vi "Initialize Subpanel Objects.vi"(8 "error in (no error)":errorcluster, 10 "SubPanelRefs":refnum<vi>[](array[refnum]), 11 "HSplittedX2 in":refnum<class "HSplittedX2.lvclass">) -> (0 "error out":errorcluster, 3 "HSplittedX2 out":refnum<class "HSplittedX2.lvclass">)   [LabVIEW 2020, in "HSplittedX2.lvlib" / "HSplittedX2.lvclass"]
uses:
  HSplittedX2.lvclass
  HSplittedX2.lvclass/HSplittedX2.ctl
  <vilib>/MGI/Panel Manager/Panel/Panel.lvlib
  <vilib>/MGI/Panel Manager/Panel/Panel/Subpanel/Subpanel.vi
  <vilib>/MGI/Panel Manager/Panel/Panel/Subpanel/Subpanel.lvclass
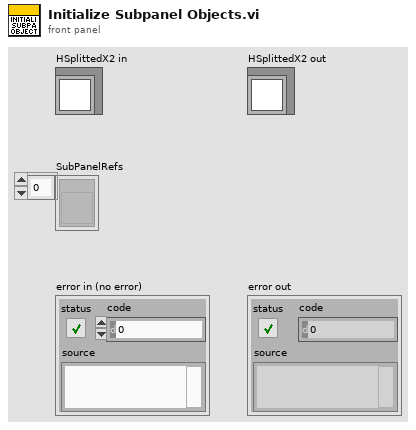
[diagram p1: front panel]
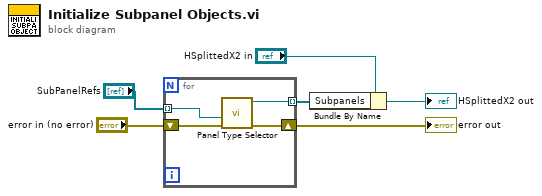
[diagram p0: block diagram]
diagram:
  n1 = for {
    tunnel: "SubPanelRefs" -> [w10] mode=indexing
    tunnel: [w9] -> w4 mode=indexing
    shift-right: [w7] -> w6
    shift-left: "error in (no error)" -> [w8]
    n2 = call-poly <vilib>:"Panel Type Selector.vi"("Error In"=w8, "Sub Panel"=w10) -> ("Error Out"=w7:errorcluster, "Subpanel Out"=w9:refnum<class "Subpanel.lvclass">)  [unwired: 8 in]
  }
  "error out" <- w6
  n3 = Bundle By Name(cluster="HSplittedX2 in", "Subpanels"=w4) -> (→"HSplittedX2 out":refnum<class "HSplittedX2.lvclass">)
